vi "acquire multi waves subvi.vi"(0 "WaveformGraph in":refnum<vi>, 1 "read buffer":string, 2 "VISA Refnum in":refnum<visa-resource-name>, 5 "error in (no error)":errorcluster) -> (7 "CH1 PROBE":string, 8 "CH1 VOLTS/DIV":string, 9 "Array":i32[][](array[numeric]), 10 "CH2 VOLTS/DIV":string, 11 "(hi.lo) 2":u16, 12 "CH1 2":string, 13 "CH2 PROBE":string, 14 "CH1":string, 15 "SEC/DIV":string, 16 "CH2 SCALE":string, 17 "CH2":string, 18 "Enum":enum16{"Idle", "Start"}(ring))   [LabVIEW 2013]
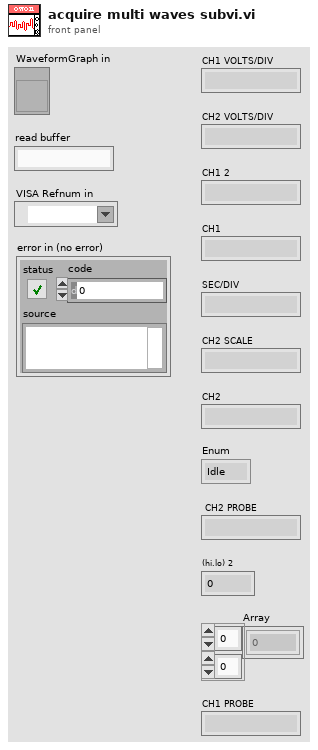
[diagram p1: front panel]
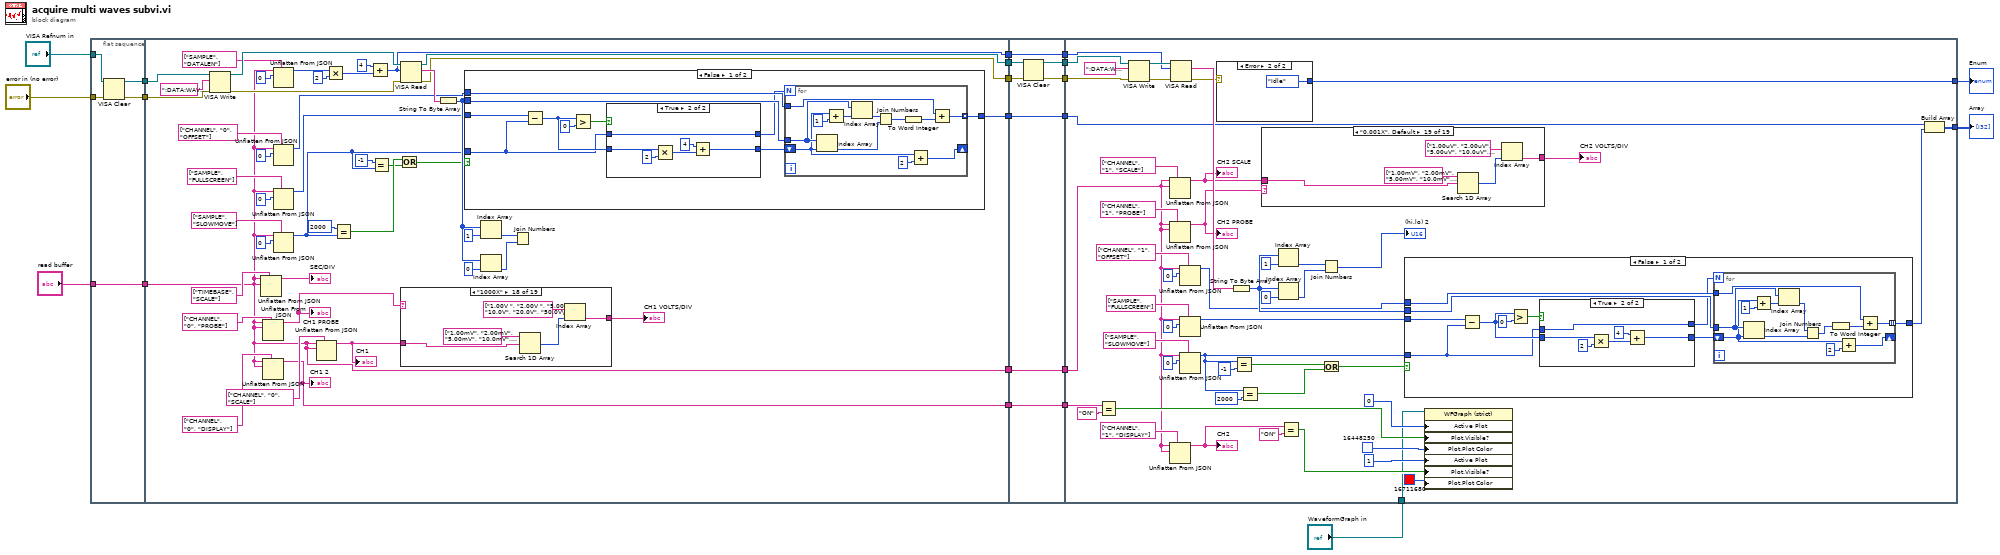
[diagram p0: block diagram]
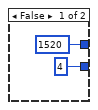
[diagram p2: hidden frame]
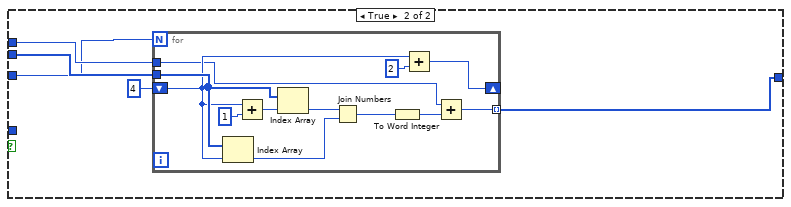
[diagram p3: hidden frame]
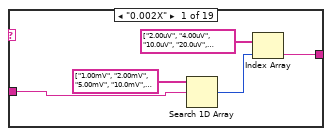
[diagram p4: hidden frame]
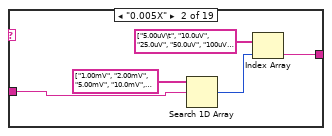
[diagram p5: hidden frame]
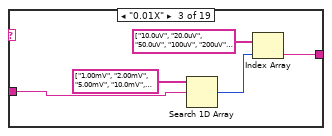
[diagram p6: hidden frame]
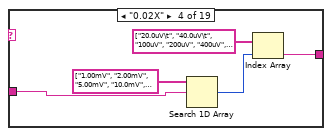
[diagram p7: hidden frame]
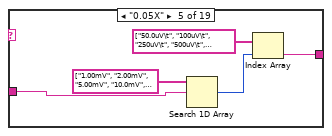
[diagram p8: hidden frame]
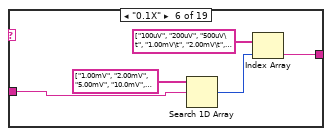
[diagram p9: hidden frame]
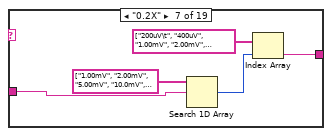
[diagram p10: hidden frame]
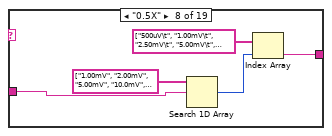
[diagram p11: hidden frame]
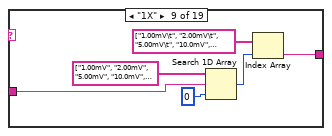
[diagram p12: hidden frame]
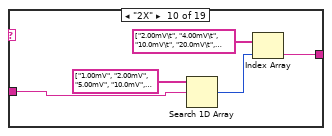
[diagram p13: hidden frame]
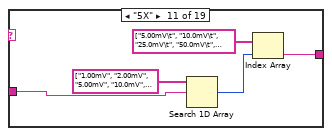
[diagram p14: hidden frame]
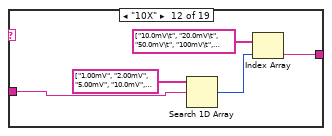
[diagram p15: hidden frame]
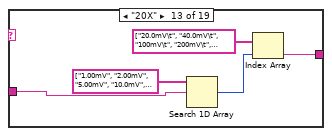
[diagram p16: hidden frame]
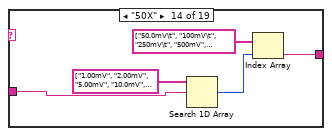
[diagram p17: hidden frame]
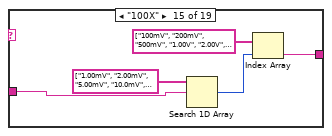
[diagram p18: hidden frame]
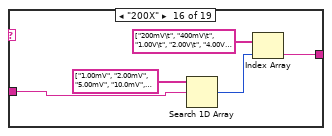
[diagram p19: hidden frame]
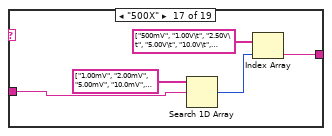
[diagram p20: hidden frame]
diagram:
  n1 = flat-sequence {
    tunnel: "read buffer" -> [w26]
    tunnel: [w25] -> w21
    tunnel: [w24] -> w20
    tunnel: [w26] -> w19
    tunnel: "VISA Refnum in" -> [w23]
    tunnel: "error in (no error)" -> [w22]
    tunnel: w21 -> [w71]
    tunnel: w20 -> [w70]
    tunnel: w19 -> [w34]
    tunnel: [w34] -> w18
    tunnel: [w49] -> w17
    tunnel: [w48] -> w16
    tunnel: [w47] -> w15
    tunnel: [w46] -> w14
    tunnel: [w36] -> w13
    tunnel: [w222] -> w12
    tunnel: w18 -> [w222]
    tunnel: w17 -> [w221]
    tunnel: w16 -> [w220]
    tunnel: [w219] -> w11
    tunnel: [w218] -> w10
    tunnel: w15 -> [w217]
    tunnel: [w217] -> w9
    tunnel: w14 -> [w216]
    tunnel: [w216] -> w8
    tunnel: [w215] -> w7
    tunnel: w13 -> [w215]
    tunnel: [w272] -> w3
    tunnel: w12 -> [w233]
    tunnel: w11 -> [w266]
    tunnel: w10 -> [w265]
    tunnel: w9 -> [w261]
    tunnel: w8 -> [w236]
    tunnel: w7 -> [w247]
    tunnel: [w224] -> w6
    tunnel: "WaveformGraph in" -> [w223]
    frame #0 {
      n2 = VISA Clear(VISA resource name=w23, error in (no error)=w22) -> (VISA resource name out=w25:refnum<visa-resource-name>, error out=w24:errorcluster)
    }
    frame #1 {
      n3 = VISA Write(VISA resource name=w71, write buffer=":DATA:WAVE:SCREEN:CH1?" ("ID Query"), error in (no error)=w70) -> (VISA resource name out=w69:refnum<visa-resource-name>, error out=w68:errorcluster)  [unwired: 1 out]
      n4 = Unflatten From JSON(path=string[] ["TIMEBASE", "SCALE"], JSON string=w34, type and defaults=w34) -> (value=→"SEC/DIV":string)  [unwired: 4 in, 1 out]
      n5 = Unflatten From JSON(path=string[] ["CHANNEL", "0", "PROBE"], JSON string=w34, type and defaults=w34) -> (value=w45:string)  [unwired: 4 in, 1 out]
      "CH1 PROBE" <- w45
      n6 = Unflatten From JSON(path=string[] ["CHANNEL", "0", "DISPLAY"], JSON string=w34, type and defaults=w34) -> (value=w36:string)  [unwired: 4 in, 1 out]
      "CH1 2" <- w36
      n7 = Unflatten From JSON(path=string[] ["SAMPLE", "DATALEN"], JSON string=w34, type and defaults=0) -> (value=w53:i32)  [unwired: 4 in, 1 out]
      n8 = Unflatten From JSON(path=string[] ["CHANNEL", "0", "OFFSET"], JSON string=w34, type and defaults=0) -> (value=w56:i32)  [unwired: 4 in, 1 out]
      n9 = Unflatten From JSON(path=string[] ["SAMPLE", "FULLSCREEN"], JSON string=w34, type and defaults=0) -> (value=w40:i32)  [unwired: 4 in, 1 out]
      n10 = Unflatten From JSON(path=string[] ["SAMPLE", "SLOWMOVE"], JSON string=w34, type and defaults=0) -> (value=w27:i32)  [unwired: 4 in, 1 out]
      n11 = Unflatten From JSON(path=string[] ["CHANNEL", "0", "SCALE"], JSON string=w34, type and defaults=w34) -> (value=w44:string)  [unwired: 4 in, 1 out]
      "CH1" <- w44
      n12 = Multiply(x=w53, y=2) -> (x*y=w51:i32)
      n13 = Equal?(x=2000, y=w27) -> (x = y?=w31:bool)
      n14 = Add(x=4, y=w51) -> (x+y=w47:i32)
      n15 = Equal?(x=-1, y=w27) -> (x = y?=w28:bool)
      n16 = Or(x=w31, y=w28) -> (x .or. y?=w32:bool)
      n17 = VISA Read(VISA resource name=w69, byte count=w47, error in (no error)=w68) -> (VISA resource name out=w49:refnum<visa-resource-name>, read buffer=w62:string, error out=w48:errorcluster)  [unwired: 1 out]
      n18 = case shown="\"1000X\"" w45 {
        tunnel: w44 -> [w122 w127 w132 w137 w142 w147 w152 w157 w162 w168 w173 w178 w183 w188 w193 w198 w203 w208 w214]
        tunnel: [w121 w126 w131 w136 w141 w146 w151 w156 w161 w167 w172 w177 w182 w187 w192 w197 w202 w207 w211] -> w43
        frame "0.002X" {
          n19 = Search 1D Array(1D array=string[] ["1.00mV", "2.00mV", "5.00mV", "10.0mV", "20.0mV", "50.0mV", "100mV", "200mV", "500mV", "1.00V", "2.00V", "5.00V", "10.0V", "20.0V"], element=w122) -> (index of element=w123:i32)  [unwired: 1 in]
          n20 = Index Array(array=string[] ["2.00uV", "4.00uV", "10.0uV", "20.0uV", "50.0uV", "100uV", "200uV", "400uV", "1.00mV", "2.00mV\t", "4.00mV", "10.0mV", "20.0mV", "40.0mV"], index=w123) -> (element=w121:string)
        }
        frame "0.005X" {
          n21 = Search 1D Array(1D array=string[] ["1.00mV", "2.00mV", "5.00mV", "10.0mV", "20.0mV", "50.0mV", "100mV", "200mV", "500mV", "1.00V", "2.00V", "5.00V", "10.0V", "20.0V"], element=w127) -> (index of element=w128:i32)  [unwired: 1 in]
          n22 = Index Array(array=string[] ["5.00uV\t", "10.0uV", "25.0uV", "50.0uV", "100uV", "250uV", "500uV", "1.00mV\t", "2.50mV", "5.00mV", "10.0mV", "25.0mV", "50.0mV", "100mV"], index=w128) -> (element=w126:string)
        }
        frame "0.01X" {
          n23 = Search 1D Array(1D array=string[] ["1.00mV", "2.00mV", "5.00mV", "10.0mV", "20.0mV", "50.0mV", "100mV", "200mV", "500mV", "1.00V", "2.00V", "5.00V", "10.0V", "20.0V"], element=w132) -> (index of element=w133:i32)  [unwired: 1 in]
          n24 = Index Array(array=string[] ["10.0uV", "20.0uV", "50.0uV", "100uV", "200uV", "500uV", "1.00mV\t", "2.00mV\t", "5.00mV", "10.0mV\t", "20.0mV\t", "50.0mV", "100mV", "200mV"], index=w133) -> (element=w131:string)
        }
        frame "0.02X" {
          n25 = Search 1D Array(1D array=string[] ["1.00mV", "2.00mV", "5.00mV", "10.0mV", "20.0mV", "50.0mV", "100mV", "200mV", "500mV", "1.00V", "2.00V", "5.00V", "10.0V", "20.0V"], element=w137) -> (index of element=w138:i32)  [unwired: 1 in]
          n26 = Index Array(array=string[] ["20.0uV\t", "40.0uV\t", "100uV", "200uV", "400uV", "1.00mV", "2.00mV", "4.00mV", "10.0mV", "20.0mV", "40.0mV", "100mV", "200mV", "400mV"], index=w138) -> (element=w136:string)
        }
        frame "0.05X" {
          n27 = Search 1D Array(1D array=string[] ["1.00mV", "2.00mV", "5.00mV", "10.0mV", "20.0mV", "50.0mV", "100mV", "200mV", "500mV", "1.00V", "2.00V", "5.00V", "10.0V", "20.0V"], element=w142) -> (index of element=w143:i32)  [unwired: 1 in]
          n28 = Index Array(array=string[] ["50.0uV\t", "100uV\t", "250uV\t", "500uV\t", "1.00mV", "2.50mV\t", "5.00mV\t", "10.0mV\t", "25.0mV", "50.0mV\t", "100mV", "250mV", "500mV", "1.00V"], index=w143) -> (element=w141:string)
        }
        frame "0.1X" {
          n29 = Search 1D Array(1D array=string[] ["1.00mV", "2.00mV", "5.00mV", "10.0mV", "20.0mV", "50.0mV", "100mV", "200mV", "500mV", "1.00V", "2.00V", "5.00V", "10.0V", "20.0V"], element=w147) -> (index of element=w148:i32)  [unwired: 1 in]
          n30 = Index Array(array=string[] ["100uV", "200uV", "500uV\t", "1.00mV\t", "2.00mV\t", "5.00mV\t", "10.0mV\t", "20.0mV\t", "50.0mV\t", "100mV", "200mV", "500mV\t", "1.00V", "2.00V"], index=w148) -> (element=w146:string)
        }
        frame "0.2X" {
          n31 = Search 1D Array(1D array=string[] ["1.00mV", "2.00mV", "5.00mV", "10.0mV", "20.0mV", "50.0mV", "100mV", "200mV", "500mV", "1.00V", "2.00V", "5.00V", "10.0V", "20.0V"], element=w152) -> (index of element=w153:i32)  [unwired: 1 in]
          n32 = Index Array(array=string[] ["200uV\t", "400uV", "1.00mV", "2.00mV", "4.00mV\t", "10.0mV", "20.0mV", "40.0mV\t", "100mV", "200mV", "400mV", "1.00V", "2.00V", "4.00V"], index=w153) -> (element=w151:string)
        }
        frame "0.5X" {
          n33 = Search 1D Array(1D array=string[] ["1.00mV", "2.00mV", "5.00mV", "10.0mV", "20.0mV", "50.0mV", "100mV", "200mV", "500mV", "1.00V", "2.00V", "5.00V", "10.0V", "20.0V"], element=w157) -> (index of element=w158:i32)  [unwired: 1 in]
          n34 = Index Array(array=string[] ["500uV\t", "1.00mV\t", "2.50mV\t", "5.00mV\t", "10.0mV\t", "25.0mV\t", "50.0mV\t", "100mV", "250mV\t", "500mV\t", "1.00V\t", "2.50V\t", "5.00V\t", "10.0V"], index=w158) -> (element=w156:string)
        }
        frame "1X" {
          n35 = Search 1D Array(1D array=string[] ["1.00mV", "2.00mV", "5.00mV", "10.0mV", "20.0mV", "50.0mV", "100mV", "200mV", "500mV", "1.00V", "2.00V", "5.00V", "10.0V", "20.0V"], element=w162, start index (0)=0 ("开始索引(0)")) -> (index of element=w163:i32)
          n36 = Index Array(array=string[] ["1.00mV\t", "2.00mV\t", "5.00mV\t", "10.0mV", "20.0mV", "50.0mV", "100mV", "200mV\t", "500mV", "1.00V\t", "2.00V", "5.00V", "10.0V", "20.0V"], index=w163) -> (element=w161:string)
        }
        frame "2X" {
          n37 = Search 1D Array(1D array=string[] ["1.00mV", "2.00mV", "5.00mV", "10.0mV", "20.0mV", "50.0mV", "100mV", "200mV", "500mV", "1.00V", "2.00V", "5.00V", "10.0V", "20.0V"], element=w168) -> (index of element=w169:i32)  [unwired: 1 in]
          n38 = Index Array(array=string[] ["2.00mV\t", "4.00mV\t", "10.0mV\t", "20.0mV\t", "40.0mV", "100mV\t", "200mV", "400mV", "1.00V\t", "2.00V", "4.00V", "10.0V", "20.0V", "40.0V"], index=w169) -> (element=w167:string)
        }
        frame "5X" {
          n39 = Search 1D Array(1D array=string[] ["1.00mV", "2.00mV", "5.00mV", "10.0mV", "20.0mV", "50.0mV", "100mV", "200mV", "500mV", "1.00V", "2.00V", "5.00V", "10.0V", "20.0V"], element=w173) -> (index of element=w174:i32)  [unwired: 1 in]
          n40 = Index Array(array=string[] ["5.00mV\t", "10.0mV\t", "25.0mV\t", "50.0mV\t", "100mV\t", "250mV\t", "500mV", "1.00V", "2.50V\t", "5.00V", "10.0V\t", "25.0V", "50.0V ", "100V"], index=w174) -> (element=w172:string)
        }
        frame "10X" {
          n41 = Search 1D Array(1D array=string[] ["1.00mV", "2.00mV", "5.00mV", "10.0mV", "20.0mV", "50.0mV", "100mV", "200mV", "500mV", "1.00V", "2.00V", "5.00V", "10.0V", "20.0V"], element=w178) -> (index of element=w179:i32)  [unwired: 1 in]
          n42 = Index Array(array=string[] ["10.0mV\t", "20.0mV\t", "50.0mV\t", "100mV\t", "200mV", "500mV\t", "1.00V", "2.00V\t", "5.00V\t", "10.0V\t", "20.0V\t", "50.0V", "100V ", "200V"], index=w179) -> (element=w177:string)
        }
        frame "20X" {
          n43 = Search 1D Array(1D array=string[] ["1.00mV", "2.00mV", "5.00mV", "10.0mV", "20.0mV", "50.0mV", "100mV", "200mV", "500mV", "1.00V", "2.00V", "5.00V", "10.0V", "20.0V"], element=w183) -> (index of element=w184:i32)  [unwired: 1 in]
          n44 = Index Array(array=string[] ["20.0mV\t", "40.0mV\t", "100mV\t", "200mV\t", "400mV", "1.00V\t", "2.00V\t", "4.00V\t", "10.0V\t", "20.0V\t", "40.0V", "100V", "200V\t", "400V"], index=w184) -> (element=w182:string)
        }
        frame "50X" {
          n45 = Search 1D Array(1D array=string[] ["1.00mV", "2.00mV", "5.00mV", "10.0mV", "20.0mV", "50.0mV", "100mV", "200mV", "500mV", "1.00V", "2.00V", "5.00V", "10.0V", "20.0V"], element=w188) -> (index of element=w189:i32)  [unwired: 1 in]
          n46 = Index Array(array=string[] ["50.0mV\t", "100mV\t", "250mV\t", "500mV", "1.00V", "2.50V\t", "5.00V\t", "10.0V\t", "25.0V\t", "50.0V\t", "100V", "250V", "500V\t", "1.00kV"], index=w189) -> (element=w187:string)
        }
        frame "100X" {
          n47 = Search 1D Array(1D array=string[] ["1.00mV", "2.00mV", "5.00mV", "10.0mV", "20.0mV", "50.0mV", "100mV", "200mV", "500mV", "1.00V", "2.00V", "5.00V", "10.0V", "20.0V"], element=w193) -> (index of element=w194:i32)  [unwired: 1 in]
          n48 = Index Array(array=string[] ["100mV", "200mV", "500mV", "1.00V", "2.00V", "5.00V", "10.0V", "20.0V", "50.0V", "100V   ", "200V", "500V", "1.00kV\t", "2.00kV"], index=w194) -> (element=w192:string)
        }
        frame "200X" {
          n49 = Search 1D Array(1D array=string[] ["1.00mV", "2.00mV", "5.00mV", "10.0mV", "20.0mV", "50.0mV", "100mV", "200mV", "500mV", "1.00V", "2.00V", "5.00V", "10.0V", "20.0V"], element=w198) -> (index of element=w199:i32)  [unwired: 1 in]
          n50 = Index Array(array=string[] ["200mV\t", "400mV\t", "1.00V\t", "2.00V\t", "4.00V\t", "10.0V\t", "20.0V\t", "40.0V\t", "100V   ", "200V    ", "400V   ", "1.00kV", "2.00kV", "4.00kV"], index=w199) -> (element=w197:string)
        }
        frame "500X" {
          n51 = Search 1D Array(1D array=string[] ["1.00mV", "2.00mV", "5.00mV", "10.0mV", "20.0mV", "50.0mV", "100mV", "200mV", "500mV", "1.00V", "2.00V", "5.00V", "10.0V", "20.0V"], element=w203) -> (index of element=w204:i32)  [unwired: 1 in]
          n52 = Index Array(array=string[] ["500mV", "1.00V\t", "2.50V\t", "5.00V\t", "10.0V\t", "25.0V", "50.0V", "100V   ", "250V\t", "500V\t    ", "1.00kV\t", "2.50kV", "5.00kV", "10.0kV"], index=w204) -> (element=w202:string)
        }
        frame "1000X" {
          n53 = Search 1D Array(1D array=string[] ["1.00mV", "2.00mV", "5.00mV", "10.0mV", "20.0mV", "50.0mV", "100mV", "200mV", "500mV", "1.00V", "2.00V", "5.00V", "10.0V", "20.0V"], element=w208) -> (index of element=w209:i32)  [unwired: 1 in]
          n54 = Index Array(array=string[] ["1.00V ", "2.00V ", "5.00V\t", "10.0V", "20.0V", "50.0V\t", "100V", "200V  ", "500V   ", "1.00kV\t   ", "2.00kV ", "5.00kV\t", "10.0kV", "20.0kV"], index=w209) -> (element=w207:string)
        }
        frame "0.001X", Default {
          n55 = Search 1D Array(1D array=string[] ["1.00mV", "2.00mV", "5.00mV", "10.0mV", "20.0mV", "50.0mV", "100mV", "200mV", "500mV", "1.00V", "2.00V", "5.00V", "10.0V", "20.0V"], element=w214) -> (index of element=w213:i32)  [unwired: 1 in]
          n56 = Index Array(array=string[] ["1.00uV", "2.00uV", "5.00uV", "10.0uV", "20.0uV", "50.0uV,\t", "100uV,\t", "200uV,\t", "500uV,\t", "1.00mV,\t", "2.00mV,\t", "5.00mV,\t", "10.0mV, ", "20.0mv"], index=w213) -> (element=w211:string)
        }
      }
      "CH1 VOLTS/DIV" <- w43
      n57 = String To Byte Array(string=w62) -> (unsigned byte array=w59:u8[])
      n58 = case shown="False" w32 {
        tunnel: w59 -> [w79 w106]
        tunnel: w56 -> [w80 w105]
        tunnel: [w81 w104] -> w46
        tunnel: w40 -> [w72 w102]
        tunnel: w27 -> [w73 _]
        frame False {
          n59 = Subtract(x=w72, y=w73) -> (x-y=w77:i32)
          n60 = Greater?(x=w77, y=0) -> (0:w78:bool)
          n61 = case shown="True" w78 {
            tunnel: [4 w88] -> w74
            tunnel: w77 -> [_ w85]
            tunnel: [1520 w84] -> w75
            tunnel: w73 -> [_ w84]
            frame False {
            }
            frame True {
              n62 = Multiply(x=w85, y=2) -> (x*y=w87:i32)
              n63 = Add(x=4, y=w87) -> (x+y=w88:i32)
            }
          }
          n64 = for {
            N: w75 -> [_]
            tunnel: w79 -> [w101]
            shift-right: [w98] -> _
            shift-left: w74 -> [w97]
            tunnel: [w95] -> w81 mode=indexing
            tunnel: w80 -> [w92]
            n65 = Index Array(array=w101, index=w97) -> (element=w93:u8)
            n66 = Add(x=w97, y=1) -> (x+y=w100:i32)
            n67 = Index Array(array=w101, index=w100) -> (element=w94:u8)
            n68 = Join Numbers(hi=w94, lo=w93) -> ((hi.lo)=w91:u16)
            n69 = To Word Integer(number=w91) -> (16bit integer=w90:i16)
            n70 = Add(x=w97, y=2) -> (x+y=w98:i32)
            n71 = Add(x=w92, y=w90) -> (x+y=w95:i32)
          }
        }
        frame True {
          n72 = for {
            N: w102 -> [_]
            tunnel: w106 -> [w118]
            shift-right: [w115] -> _
            shift-left: 4 -> [w114]
            tunnel: [w112] -> w104 mode=indexing
            tunnel: w105 -> [w109]
            n73 = Index Array(array=w118, index=w114) -> (element=w110:u8)
            n74 = Add(x=w114, y=1) -> (x+y=w117:i32)
            n75 = Index Array(array=w118, index=w117) -> (element=w111:u8)
            n76 = Join Numbers(hi=w111, lo=w110) -> ((hi.lo)=w108:u16)
            n77 = To Word Integer(number=w108) -> (16bit integer=w107:i16)
            n78 = Add(x=w114, y=2) -> (x+y=w115:i32)
            n79 = Add(x=w109, y=w107) -> (x+y=w112:i32)
          }
        }
      }
      n80 = Index Array(array=w59, index=1) -> (element=w64:u8)
      n81 = Index Array(array=w59, index=0) -> (element=w63:u8)
      n82 = Join Numbers(hi=w64, lo=w63) -> ()  [unwired: 1 out]
    }
    frame #2 {
      n83 = VISA Clear(VISA resource name=w221, error in (no error)=w220) -> (VISA resource name out=w219:refnum<visa-resource-name>, error out=w218:errorcluster)
    }
    frame #3 {
      n84 = Equal?(x=w247, y="ON") -> (x = y?=w243:bool)
      n85 = VISA Write(VISA resource name=w266, write buffer=":DATA:WAVE:SCREEN:CH2?" ("ID Query"), error in (no error)=w265) -> (VISA resource name out=w263:refnum<visa-resource-name>, error out=w262:errorcluster)  [unwired: 1 out]
      n86 = Unflatten From JSON(path=string[] ["CHANNEL", "1", "SCALE"], JSON string=w233, type and defaults=w233) -> (value=w249:string)  [unwired: 4 in, 1 out]
      "CH2 SCALE" <- w249
      n87 = Unflatten From JSON(path=string[] ["CHANNEL", "1", "PROBE"], JSON string=w233, type and defaults=w233) -> (value=w250:string)  [unwired: 4 in, 1 out]
      "CH2 PROBE" <- w250
      n88 = Unflatten From JSON(path=string[] ["CHANNEL", "1", "DISPLAY"], JSON string=w233, type and defaults=w233) -> (value=w245:string)  [unwired: 4 in, 1 out]
      "CH2" <- w245
      n89 = VISA Read(VISA resource name=w263, byte count=w261, error in (no error)=w262) -> (read buffer=w254:string, error out=w251:errorcluster)  [unwired: 2 out]
      n90 = Unflatten From JSON(path=string[] ["CHANNEL", "1", "OFFSET"], JSON string=w233, type and defaults=0) -> (value=w253:i32)  [unwired: 4 in, 1 out]
      n91 = Unflatten From JSON(path=string[] ["SAMPLE", "FULLSCREEN"], JSON string=w233, type and defaults=0) -> (value=w232:i32)  [unwired: 4 in, 1 out]
      n92 = Unflatten From JSON(path=string[] ["SAMPLE", "SLOWMOVE"], JSON string=w233, type and defaults=0) -> (value=w226:i32)  [unwired: 4 in, 1 out]
      n93 = case shown="Error" w251 {
        tunnel: [enum16{"Idle", "Start"}."Start" enum16{"Idle", "Start"}."Idle"] -> w272
        frame No Error {
        }
        frame Error {
        }
      }
      n94 = String To Byte Array(string=w254) -> (unsigned byte array=w256:u8[])
      n95 = Equal?(x=w226, y=-1) -> (x = y?=w229:bool)
      n96 = Equal?(x=w226, y=2000) -> (x = y?=w225:bool)
      n97 = case shown="\"0.001X\", Default" w250 {
        tunnel: w249 -> [w323 w328 w333 w338 w343 w348 w353 w358 w363 w369 w374 w379 w384 w389 w394 w399 w404 w409 w415]
        tunnel: [w322 w327 w332 w337 w342 w347 w352 w357 w362 w368 w373 w378 w383 w388 w393 w398 w403 w408 w412] -> w248
        frame "0.002X" {
          n98 = Search 1D Array(1D array=string[] ["1.00mV", "2.00mV", "5.00mV", "10.0mV", "20.0mV", "50.0mV", "100mV", "200mV", "500mV", "1.00V", "2.00V", "5.00V", "10.0V", "20.0V"], element=w323) -> (index of element=w324:i32)  [unwired: 1 in]
          n99 = Index Array(array=string[] ["2.00uV", "4.00uV", "10.0uV", "20.0uV", "50.0uV", "100uV", "200uV", "400uV", "1.00mV", "2.00mV\t", "4.00mV", "10.0mV", "20.0mV", "40.0mV"], index=w324) -> (element=w322:string)
        }
        frame "0.005X" {
          n100 = Search 1D Array(1D array=string[] ["1.00mV", "2.00mV", "5.00mV", "10.0mV", "20.0mV", "50.0mV", "100mV", "200mV", "500mV", "1.00V", "2.00V", "5.00V", "10.0V", "20.0V"], element=w328) -> (index of element=w329:i32)  [unwired: 1 in]
          n101 = Index Array(array=string[] ["5.00uV\t", "10.0uV", "25.0uV", "50.0uV", "100uV", "250uV", "500uV", "1.00mV\t", "2.50mV", "5.00mV", "10.0mV", "25.0mV", "50.0mV", "100mV"], index=w329) -> (element=w327:string)
        }
        frame "0.01X" {
          n102 = Search 1D Array(1D array=string[] ["1.00mV", "2.00mV", "5.00mV", "10.0mV", "20.0mV", "50.0mV", "100mV", "200mV", "500mV", "1.00V", "2.00V", "5.00V", "10.0V", "20.0V"], element=w333) -> (index of element=w334:i32)  [unwired: 1 in]
          n103 = Index Array(array=string[] ["10.0uV", "20.0uV", "50.0uV", "100uV", "200uV", "500uV", "1.00mV\t", "2.00mV\t", "5.00mV", "10.0mV\t", "20.0mV\t", "50.0mV", "100mV", "200mV"], index=w334) -> (element=w332:string)
        }
        frame "0.02X" {
          n104 = Search 1D Array(1D array=string[] ["1.00mV", "2.00mV", "5.00mV", "10.0mV", "20.0mV", "50.0mV", "100mV", "200mV", "500mV", "1.00V", "2.00V", "5.00V", "10.0V", "20.0V"], element=w338) -> (index of element=w339:i32)  [unwired: 1 in]
          n105 = Index Array(array=string[] ["20.0uV\t", "40.0uV\t", "100uV", "200uV", "400uV", "1.00mV", "2.00mV", "4.00mV", "10.0mV", "20.0mV", "40.0mV", "100mV", "200mV", "400mV"], index=w339) -> (element=w337:string)
        }
        frame "0.05X" {
          n106 = Search 1D Array(1D array=string[] ["1.00mV", "2.00mV", "5.00mV", "10.0mV", "20.0mV", "50.0mV", "100mV", "200mV", "500mV", "1.00V", "2.00V", "5.00V", "10.0V", "20.0V"], element=w343) -> (index of element=w344:i32)  [unwired: 1 in]
          n107 = Index Array(array=string[] ["50.0uV\t", "100uV\t", "250uV\t", "500uV\t", "1.00mV", "2.50mV\t", "5.00mV\t", "10.0mV\t", "25.0mV", "50.0mV\t", "100mV", "250mV", "500mV", "1.00V"], index=w344) -> (element=w342:string)
        }
        frame "0.1X" {
          n108 = Search 1D Array(1D array=string[] ["1.00mV", "2.00mV", "5.00mV", "10.0mV", "20.0mV", "50.0mV", "100mV", "200mV", "500mV", "1.00V", "2.00V", "5.00V", "10.0V", "20.0V"], element=w348) -> (index of element=w349:i32)  [unwired: 1 in]
          n109 = Index Array(array=string[] ["100uV", "200uV", "500uV\t", "1.00mV\t", "2.00mV\t", "5.00mV\t", "10.0mV\t", "20.0mV\t", "50.0mV\t", "100mV", "200mV", "500mV\t", "1.00V", "2.00V"], index=w349) -> (element=w347:string)
        }
        frame "0.2X" {
          n110 = Search 1D Array(1D array=string[] ["1.00mV", "2.00mV", "5.00mV", "10.0mV", "20.0mV", "50.0mV", "100mV", "200mV", "500mV", "1.00V", "2.00V", "5.00V", "10.0V", "20.0V"], element=w353) -> (index of element=w354:i32)  [unwired: 1 in]
          n111 = Index Array(array=string[] ["200uV\t", "400uV", "1.00mV", "2.00mV", "4.00mV\t", "10.0mV", "20.0mV", "40.0mV\t", "100mV", "200mV", "400mV", "1.00V", "2.00V", "4.00V"], index=w354) -> (element=w352:string)
        }
        frame "0.5X" {
          n112 = Search 1D Array(1D array=string[] ["1.00mV", "2.00mV", "5.00mV", "10.0mV", "20.0mV", "50.0mV", "100mV", "200mV", "500mV", "1.00V", "2.00V", "5.00V", "10.0V", "20.0V"], element=w358) -> (index of element=w359:i32)  [unwired: 1 in]
          n113 = Index Array(array=string[] ["500uV\t", "1.00mV\t", "2.50mV\t", "5.00mV\t", "10.0mV\t", "25.0mV\t", "50.0mV\t", "100mV", "250mV\t", "500mV\t", "1.00V\t", "2.50V\t", "5.00V\t", "10.0V"], index=w359) -> (element=w357:string)
        }
        frame "1X" {
          n114 = Search 1D Array(1D array=string[] ["1.00mV", "2.00mV", "5.00mV", "10.0mV", "20.0mV", "50.0mV", "100mV", "200mV", "500mV", "1.00V", "2.00V", "5.00V", "10.0V", "20.0V"], element=w363, start index (0)=0 ("开始索引(0)")) -> (index of element=w364:i32)
          n115 = Index Array(array=string[] ["1.00mV\t", "2.00mV\t", "5.00mV\t", "10.0mV", "20.0mV", "50.0mV", "100mV", "200mV\t", "500mV", "1.00V\t", "2.00V", "5.00V", "10.0V", "20.0V"], index=w364) -> (element=w362:string)
        }
        frame "2X" {
          n116 = Search 1D Array(1D array=string[] ["1.00mV", "2.00mV", "5.00mV", "10.0mV", "20.0mV", "50.0mV", "100mV", "200mV", "500mV", "1.00V", "2.00V", "5.00V", "10.0V", "20.0V"], element=w369) -> (index of element=w370:i32)  [unwired: 1 in]
          n117 = Index Array(array=string[] ["2.00mV\t", "4.00mV\t", "10.0mV\t", "20.0mV\t", "40.0mV", "100mV\t", "200mV", "400mV", "1.00V\t", "2.00V", "4.00V", "10.0V", "20.0V", "40.0V"], index=w370) -> (element=w368:string)
        }
        frame "5X" {
          n118 = Search 1D Array(1D array=string[] ["1.00mV", "2.00mV", "5.00mV", "10.0mV", "20.0mV", "50.0mV", "100mV", "200mV", "500mV", "1.00V", "2.00V", "5.00V", "10.0V", "20.0V"], element=w374) -> (index of element=w375:i32)  [unwired: 1 in]
          n119 = Index Array(array=string[] ["5.00mV\t", "10.0mV\t", "25.0mV\t", "50.0mV\t", "100mV\t", "250mV\t", "500mV", "1.00V", "2.50V\t", "5.00V", "10.0V\t", "25.0V", "50.0V ", "100V"], index=w375) -> (element=w373:string)
        }
        frame "10X" {
          n120 = Search 1D Array(1D array=string[] ["1.00mV", "2.00mV", "5.00mV", "10.0mV", "20.0mV", "50.0mV", "100mV", "200mV", "500mV", "1.00V", "2.00V", "5.00V", "10.0V", "20.0V"], element=w379) -> (index of element=w380:i32)  [unwired: 1 in]
          n121 = Index Array(array=string[] ["10.0mV\t", "20.0mV\t", "50.0mV\t", "100mV\t", "200mV", "500mV\t", "1.00V", "2.00V\t", "5.00V\t", "10.0V\t", "20.0V\t", "50.0V", "100V ", "200V"], index=w380) -> (element=w378:string)
        }
        frame "20X" {
          n122 = Search 1D Array(1D array=string[] ["1.00mV", "2.00mV", "5.00mV", "10.0mV", "20.0mV", "50.0mV", "100mV", "200mV", "500mV", "1.00V", "2.00V", "5.00V", "10.0V", "20.0V"], element=w384) -> (index of element=w385:i32)  [unwired: 1 in]
          n123 = Index Array(array=string[] ["20.0mV\t", "40.0mV\t", "100mV\t", "200mV\t", "400mV", "1.00V\t", "2.00V\t", "4.00V\t", "10.0V\t", "20.0V\t", "40.0V", "100V", "200V\t", "400V"], index=w385) -> (element=w383:string)
        }
        frame "50X" {
          n124 = Search 1D Array(1D array=string[] ["1.00mV", "2.00mV", "5.00mV", "10.0mV", "20.0mV", "50.0mV", "100mV", "200mV", "500mV", "1.00V", "2.00V", "5.00V", "10.0V", "20.0V"], element=w389) -> (index of element=w390:i32)  [unwired: 1 in]
          n125 = Index Array(array=string[] ["50.0mV\t", "100mV\t", "250mV\t", "500mV", "1.00V", "2.50V\t", "5.00V\t", "10.0V\t", "25.0V\t", "50.0V\t", "100V", "250V", "500V\t", "1.00kV"], index=w390) -> (element=w388:string)
        }
        frame "100X" {
          n126 = Search 1D Array(1D array=string[] ["1.00mV", "2.00mV", "5.00mV", "10.0mV", "20.0mV", "50.0mV", "100mV", "200mV", "500mV", "1.00V", "2.00V", "5.00V", "10.0V", "20.0V"], element=w394) -> (index of element=w395:i32)  [unwired: 1 in]
          n127 = Index Array(array=string[] ["100mV", "200mV", "500mV", "1.00V", "2.00V", "5.00V", "10.0V", "20.0V", "50.0V", "100V   ", "200V", "500V", "1.00kV\t", "2.00kV"], index=w395) -> (element=w393:string)
        }
        frame "200X" {
          n128 = Search 1D Array(1D array=string[] ["1.00mV", "2.00mV", "5.00mV", "10.0mV", "20.0mV", "50.0mV", "100mV", "200mV", "500mV", "1.00V", "2.00V", "5.00V", "10.0V", "20.0V"], element=w399) -> (index of element=w400:i32)  [unwired: 1 in]
          n129 = Index Array(array=string[] ["200mV\t", "400mV\t", "1.00V\t", "2.00V\t", "4.00V\t", "10.0V\t", "20.0V\t", "40.0V\t", "100V   ", "200V    ", "400V   ", "1.00kV", "2.00kV", "4.00kV"], index=w400) -> (element=w398:string)
        }
        frame "500X" {
          n130 = Search 1D Array(1D array=string[] ["1.00mV", "2.00mV", "5.00mV", "10.0mV", "20.0mV", "50.0mV", "100mV", "200mV", "500mV", "1.00V", "2.00V", "5.00V", "10.0V", "20.0V"], element=w404) -> (index of element=w405:i32)  [unwired: 1 in]
          n131 = Index Array(array=string[] ["500mV", "1.00V\t", "2.50V\t", "5.00V\t", "10.0V\t", "25.0V", "50.0V", "100V   ", "250V\t", "500V\t    ", "1.00kV\t", "2.50kV", "5.00kV", "10.0kV"], index=w405) -> (element=w403:string)
        }
        frame "1000X" {
          n132 = Search 1D Array(1D array=string[] ["1.00mV", "2.00mV", "5.00mV", "10.0mV", "20.0mV", "50.0mV", "100mV", "200mV", "500mV", "1.00V", "2.00V", "5.00V", "10.0V", "20.0V"], element=w409) -> (index of element=w410:i32)  [unwired: 1 in]
          n133 = Index Array(array=string[] ["1.00V ", "2.00V ", "5.00V\t", "10.0V", "20.0V", "50.0V\t", "100V", "200V  ", "500V   ", "1.00kV\t   ", "2.00kV ", "5.00kV\t", "10.0kV", "20.0kV"], index=w410) -> (element=w408:string)
        }
        frame "0.001X", Default {
          n134 = Search 1D Array(1D array=string[] ["1.00mV", "2.00mV", "5.00mV", "10.0mV", "20.0mV", "50.0mV", "100mV", "200mV", "500mV", "1.00V", "2.00V", "5.00V", "10.0V", "20.0V"], element=w415) -> (index of element=w414:i32)  [unwired: 1 in]
          n135 = Index Array(array=string[] ["1.00uV", "2.00uV", "5.00uV", "10.0uV", "20.0uV", "50.0uV,\t", "100uV,\t", "200uV,\t", "500uV,\t", "1.00mV,\t", "2.00mV,\t", "5.00mV,\t", "10.0mV, ", "20.0mv"], index=w414) -> (element=w412:string)
        }
      }
      "CH2 VOLTS/DIV" <- w248
      n136 = Index Array(array=w256, index=1) -> (element=w258:u8)
      n137 = Index Array(array=w256, index=0) -> (element=w257:u8)
      n138 = Equal?(x=w245, y="ON") -> (x = y?=w230:bool)
      n139 = Join Numbers(hi=w258, lo=w257) -> ((hi.lo)=→"(hi.lo) 2":u16)
      n140 = Or(x=w229, y=w225) -> (x .or. y?=w231:bool)
      n141 = case shown="False" w231 {
        tunnel: w256 -> [w281 w307]
        tunnel: w253 -> [w280 w306]
        tunnel: [w282 w305] -> w252
        tunnel: w232 -> [w275 w303]
        tunnel: w226 -> [w276 _]
        frame False {
          n142 = Subtract(x=w275, y=w276) -> (x-y=w278:i32)
          n143 = Greater?(x=w278, y=0) -> (0:w277:bool)
          n144 = case shown="True" w277 {
            tunnel: [4 w289] -> w273
            tunnel: w278 -> [_ w286]
            tunnel: [1520 w285] -> w274
            tunnel: w276 -> [_ w285]
            frame False {
            }
            frame True {
              n145 = Multiply(x=w286, y=2) -> (x*y=w288:i32)
              n146 = Add(x=4, y=w288) -> (x+y=w289:i32)
            }
          }
          n147 = for {
            N: w274 -> [_]
            tunnel: w281 -> [w302]
            shift-right: [w299] -> _
            shift-left: w273 -> [w298]
            tunnel: [w296] -> w282 mode=indexing
            tunnel: w280 -> [w293]
            n148 = Index Array(array=w302, index=w298) -> (element=w294:u8)
            n149 = Add(x=w298, y=1) -> (x+y=w301:i32)
            n150 = Index Array(array=w302, index=w301) -> (element=w295:u8)
            n151 = Join Numbers(hi=w295, lo=w294) -> ((hi.lo)=w292:u16)
            n152 = To Word Integer(number=w292) -> (16bit integer=w291:i16)
            n153 = Add(x=w298, y=2) -> (x+y=w299:i32)
            n154 = Add(x=w293, y=w291) -> (x+y=w296:i32)
          }
        }
        frame True {
          n155 = for {
            N: w303 -> [_]
            tunnel: w307 -> [w319]
            shift-right: [w316] -> _
            shift-left: 4 -> [w315]
            tunnel: [w313] -> w305 mode=indexing
            tunnel: w306 -> [w310]
            n156 = Index Array(array=w319, index=w315) -> (element=w311:u8)
            n157 = Add(x=w315, y=1) -> (x+y=w318:i32)
            n158 = Index Array(array=w319, index=w318) -> (element=w312:u8)
            n159 = Join Numbers(hi=w312, lo=w311) -> ((hi.lo)=w309:u16)
            n160 = To Word Integer(number=w309) -> (16bit integer=w308:i16)
            n161 = Add(x=w315, y=2) -> (x+y=w316:i32)
            n162 = Add(x=w310, y=w308) -> (x+y=w313:i32)
          }
        }
      }
      n163 = property on="Property Node" class="WFGraph (strict)"(reference=w223, "Active Plot"=u32 0 ("活动曲线"), "Plot.Visible?"=w243, "Plot.Plot Color"=u32 16448250, "Active Plot"=u32 1 ("活动曲线"), "Plot.Visible?"=w230, "Plot.Plot Color"=u32 16711680) -> ()  [unwired: 1 in, 2 out]
      n164 = Build Array(w236, w252) -> (w224:i32[][])
    }
  }
  "Array" <- w6
  "Enum" <- w3
